vi "Lab Arreglos-2.vi"() -> ()   [LabVIEW 2018]
panel:
  out "Array":sgl[][](array[numeric])
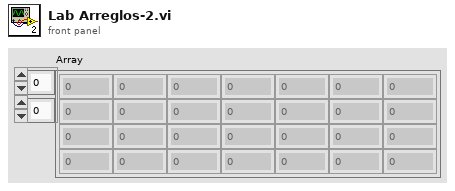
[diagram p1: front panel]
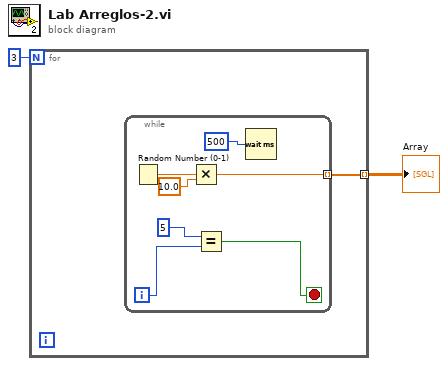
[diagram p0: block diagram]
diagram:
  n1 = for {
    N: 3 -> [_]
    tunnel: [w3] -> w2 mode=indexing
    n2 = while {
      tunnel: [w8] -> w3 mode=indexing
      i -> [w10]
      stop <- w7 stop-if-true
      n3 = Random Number (0-1)() -> (number: 0 to 1=w5:dbl)
      n4 = Multiply(x=w5, y=10.0) -> (x*y=w8:dbl)
      n5 = Equal?(x=5, y=w10) -> (x = y?=w7:bool)
      n6 = Wait (ms)(milliseconds to wait=u32 500) -> ()  [unwired: 1 out]
    }
  }
  "Array" <- w2
